vi "int2.vi"() -> ()   [LabVIEW 2017]
uses:
  <vilib>/picture/3D Picture Control/NI_3D Picture Control.lvlib
panel:
  in  "Rotación":dbl[][](array[numeric])=[[1.0, 1.0, 1.0, 1.0]]
  in  "Translación":dbl[][](array[numeric])=[[1.0, 1.0, 1.0]]
  in  "Escala":dbl[][](array[numeric])=[[1.0, 1.0, 1.0]]
  out "Archivos":i32
  out "3D Picture":refnum<vi>(3d-picture)
  in  "Stop Button":bool
  in  "Objetos":path
  in  "Mundo":path
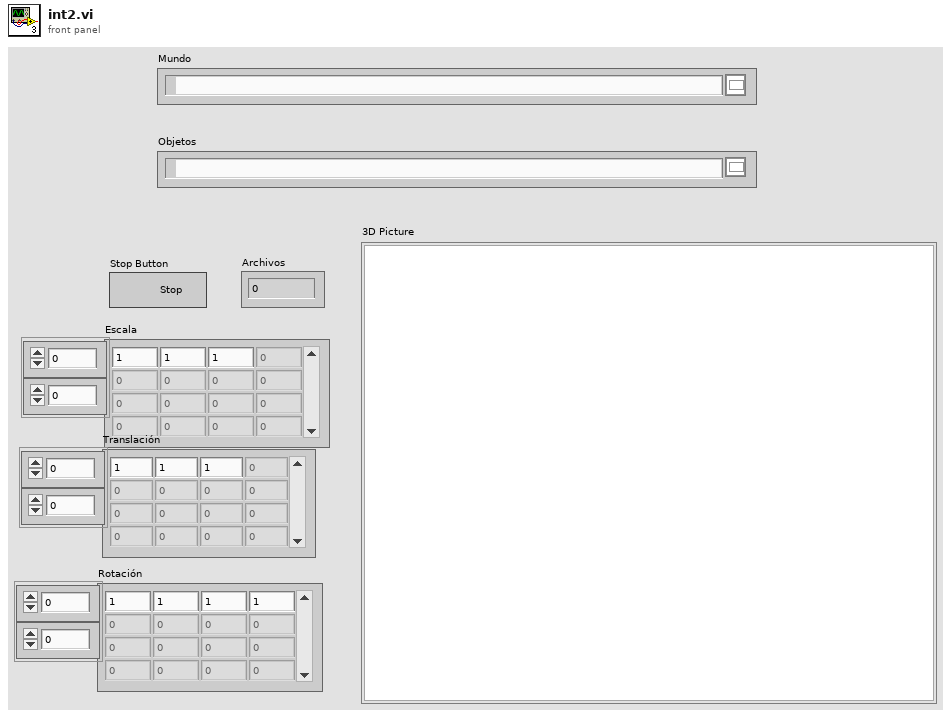
[diagram p1: front panel]
types:
  T1 = enum16{"open", "replace", "create", "open or create", "replace or create", "replace or create with confirmation"}
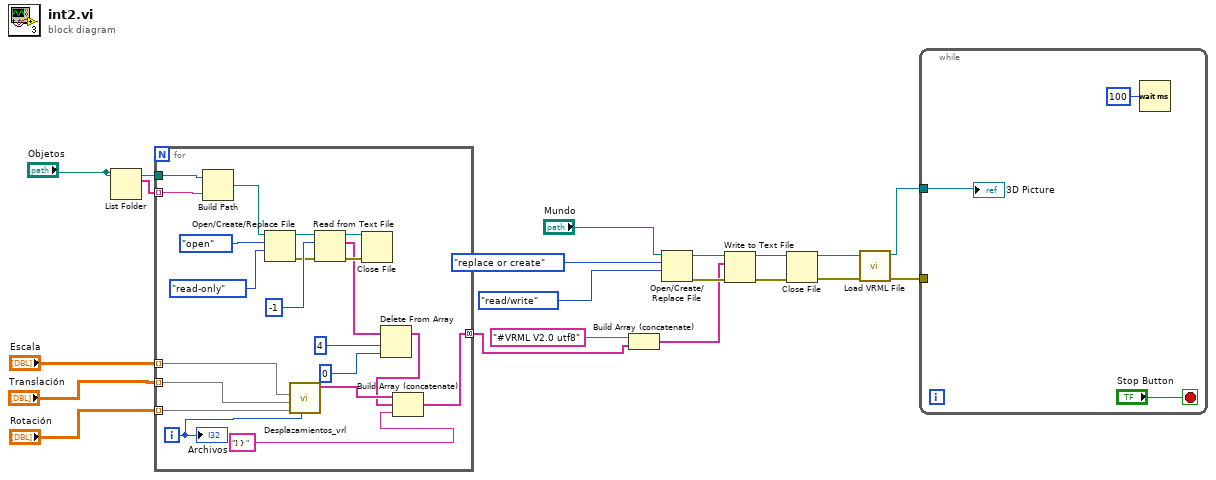
[diagram p0: block diagram]
diagram:
  n1 = List Folder(path="Objetos") -> (filenames=w12:string[])  [unwired: 3 in, 3 out]
  n2 = for {
    tunnel: w12 -> [w40] mode=indexing
    tunnel: "Objetos" -> [w39]
    tunnel: [w23] -> w5 mode=concatenating
    tunnel: "Escala" -> [w27] mode=indexing
    tunnel: "Translación" -> [w26] mode=indexing
    tunnel: "Rotación" -> [w25] mode=indexing
    i -> [w24]
    n3 = Build Path(base path=w39, name or relative path=w40) -> (appended path=w38:path)
    n4 = Open/Create/Replace File(file path (use dialog)=w38, operation (0:open)=T1."open", access (0:read/write)=enum16{"read/write", "read-only", "write-only"}."read-only") -> (refnum out=w35:refnum<file>, error out=w33:errorcluster)  [unwired: 3 in, 1 out]
    n5 = call "Desplazamientos_vrl.vi"("Indice"=w24, "Rotacion"=w25, "Translacion"=w26, "Escala"=w27) -> ("Salida"=w21:string[])  [unwired: 7 in]
    n6 = Read from Text File(file (use dialog)=w35, count=-1, error in=w33) -> (refnum out=w31:refnum<file>, text=w28:string[], error out=w32:errorcluster)  [unwired: 1 in, 1 out]
    n7 = Close File(refnum=w31, error in=w32) -> ()  [unwired: 2 out]
    n8 = Delete From Array(array=w28, length=4, index=0) -> (array with subset deleted=w20:string[])  [unwired: 1 out]
    n9 = Build Array (concatenate)(w21, w20, "] } ") -> (w23:string[])
    "Archivos" <- w24
  }
  n10 = Build Array (concatenate)("#VRML V2.0 utf8", w5) -> (w4:string[])
  n11 = Open/Create/Replace File(file path (use dialog)="Mundo", operation (0:open)=T1."replace or create", access (0:read/write)=enum16{"read/write", "read-only", "write-only"}."read/write") -> (refnum out=w16:refnum<file>, error out=w15:errorcluster)  [unwired: 3 in, 1 out]
  n12 = Write to Text File(file (use dialog)=w16, text=w4, error in=w15) -> (refnum out=w13:refnum<file>, error out=w14:errorcluster)  [unwired: 1 in, 1 out]
  n13 = Close File(refnum=w13, error in=w14) -> (path=w10:path, error out=w9:errorcluster)
  n14 = call <vilib>:"Load VRML File.vi"("error in"=w9, "Path"=w10) -> ("error out"=w7:errorcluster, "Scene:Read Scene File"=w8:refnum<vi>)  [unwired: 8 in]
  n15 = while {
    tunnel: w8 -> [w41]
    tunnel: w7 -> [_]
    stop <- "Stop Button" stop-if-true
    n16 = Wait (ms)(milliseconds to wait=u32 100) -> ()  [unwired: 1 out]
    "3D Picture" <- w41
  }
